vi "Attacked.vi"(9 "Team In":refnum<class "Team.lvclass">, 10 "Attacked Info":T1, 11 "MySquare in":refnum<class "MySquare.lvclass">) -> (1 "Team":refnum<class "Team.lvclass">, 3 "MySquare out":refnum<class "MySquare.lvclass">)   [LabVIEW 2020, in "Galaxy.lvlib" / "MySquare.lvclass"]
uses:
  MySquare.lvclass
  MySquare.lvclass/MySquare.ctl
  SquareBattle/Attacked Info.ctl
  SquareBattle/SquareBattle.lvlib
  SquareBattle/Team/Team.lvclass
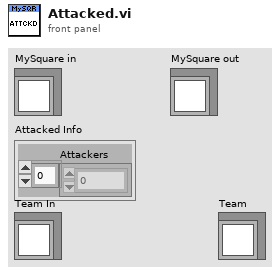
[diagram p1: front panel]
types:
  T1 = typedef "SquareBattle.lvlib/Attacked Info.ctl" = cluster{"Attackers":i32[]}
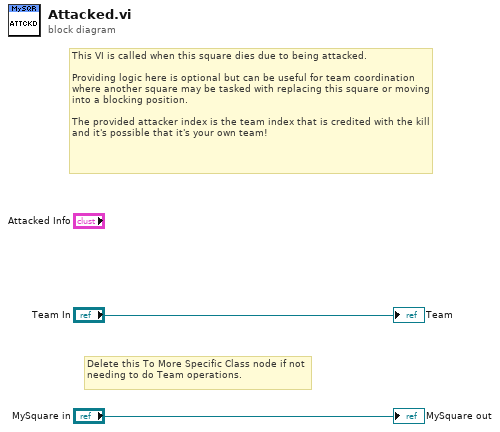
[diagram p0: block diagram]
diagram:
  # "Delete this To More Specific Class node if not needing to do Team operations."
  # "This VI is called when this square dies due to being attacked.\n\nProviding logic here is optional but can be useful for team coordination where another square may be tasked with replacing this square or moving into a blocking position.\n\nThe provided attacker index is the team index that is credited with the kill and it's possible that it's your own team!"
  "MySquare out" <- "MySquare in"
  "Team" <- "Team In"
